vi "Elevator Control PID.vi"(8 "Settings":T4={"min speed"=0.05, "Position Max"=60.0, "gravity"=0.05, "PID Constants"={"P Gain"=0.2, "I Gain"=0.0, "D Gain"=0.2, "F Gain"=0.0, "I Zone"=0.0, "Min Output"=-1.0, "Max Output"=1.0}, "SM Params"={"Max Velocity"=2000.0, "Max Acceleration"=1500.0, "Minimum Velocity Output"=0.0, "Allowed Closed Loop Error"=0.0}} {"gravity" format="%#_13g"; "Position Max" format="%#_13g"; "min speed" format="%#_13g"}, 9 "Manual":bool, 10 "Setpoint":dbl, 11 "Controller In":T6={"Setpoint"=0.0, "Output"=0.0, "DriveMotor1"={"DeviceStatus"={"status"=FALSE, "code"=0, "source"=""}, "Type"=enum."PWM", "PWM"={"PWM Channel"=enum."Invalid", "DeadBand"={"Name"="", "maxPositivePwm"=0, "minPositivePwm"=0, "centerPwm"=0, "maxNegativePwm"=0, "minNegativePwm"=0, "angularRange"=0}}, "CAN"={"Device Number"=0, "SetOutput VI Ref"=variant(enum8{"Percent VBus", "Current", "Speed", "Position", "Voltage"} enum."Percent VBus"), "GetOutput VI Ref"=variant(refnum<k1> refnum), "Enable VI Ref"=variant(dbl 12.0), "Disable VI Ref"=variant(enum8{"Percent VBus", "Speed", "Position", "Slave", "Unchanged / Invalid"} enum."Percent VBus"), "Data"=variant(enum16{"Controller 1"} enum."Controller 1")}, "Invert"=FALSE, "DIO PWM"={"PWM \"Enable\" Channel"=enum."Invalid", "DIOChannel"=enum."Invalid", "PWM Rate"=0.0}}, "Is Done Moving?"=FALSE}) -> (0 "Switches":T3, 1 "Path is Done?":bool, 2 "PID Chart":T2(graph), 3 "Controller out":T6={"Setpoint"=0.0, "Output"=0.0, "DriveMotor1"={"DeviceStatus"={"status"=FALSE, "code"=0, "source"=""}, "Type"=enum."PWM", "PWM"={"PWM Channel"=enum."Invalid", "DeadBand"={"Name"="", "maxPositivePwm"=0, "minPositivePwm"=0, "centerPwm"=0, "maxNegativePwm"=0, "minNegativePwm"=0, "angularRange"=0}}, "CAN"={"Device Number"=0, "SetOutput VI Ref"=variant(enum8{"Percent VBus", "Current", "Speed", "Position", "Voltage"} enum."Percent VBus"), "GetOutput VI Ref"=variant(refnum<k1> refnum), "Enable VI Ref"=variant(dbl 12.0), "Disable VI Ref"=variant(enum8{"Percent VBus", "Speed", "Position", "Slave", "Unchanged / Invalid"} enum."Percent VBus"), "Data"=variant(enum16{"Controller 1"} enum."Controller 1")}, "Invert"=FALSE, "DIO PWM"={"PWM \"Enable\" Channel"=enum."Invalid", "DIOChannel"=enum."Invalid", "PWM Rate"=0.0}}, "Is Done Moving?"=FALSE})   [LabVIEW 2018]
uses:
  Typedef/Controller Data.ctl
  <vilib>/Rock Robotics/WPI/MotorControl/WPI_MotorControlDeviceRef.ctl
  <vilib>/Rock Robotics/WPI/MotorControl/WPI_MotorControlType.ctl
  <vilib>/Rock Robotics/SystemInterfaces/DIO/FPGA_DIOPWMChannel.ctl
  <vilib>/Rock Robotics/WPI/PWM/WPI_PWMDeadband.ctl
  <vilib>/Rock Robotics/SystemInterfaces/DIO/FPGA_DIOChannel.ctl
  Typedef/Elevator Settings.ctl
  <vilib>/Rock Robotics/WPI/ThirdParty/REV Robotics/SPARK MAX/Typedef/Spark MAX Smart Motion Parameters.ctl
  <vilib>/Rock Robotics/WPI/ThirdParty/REV Robotics/SPARK MAX/Typedef/Spark MAX Control Type.ctl
panel:
  out "Waveform Chart":T1(graph)
  # "s"
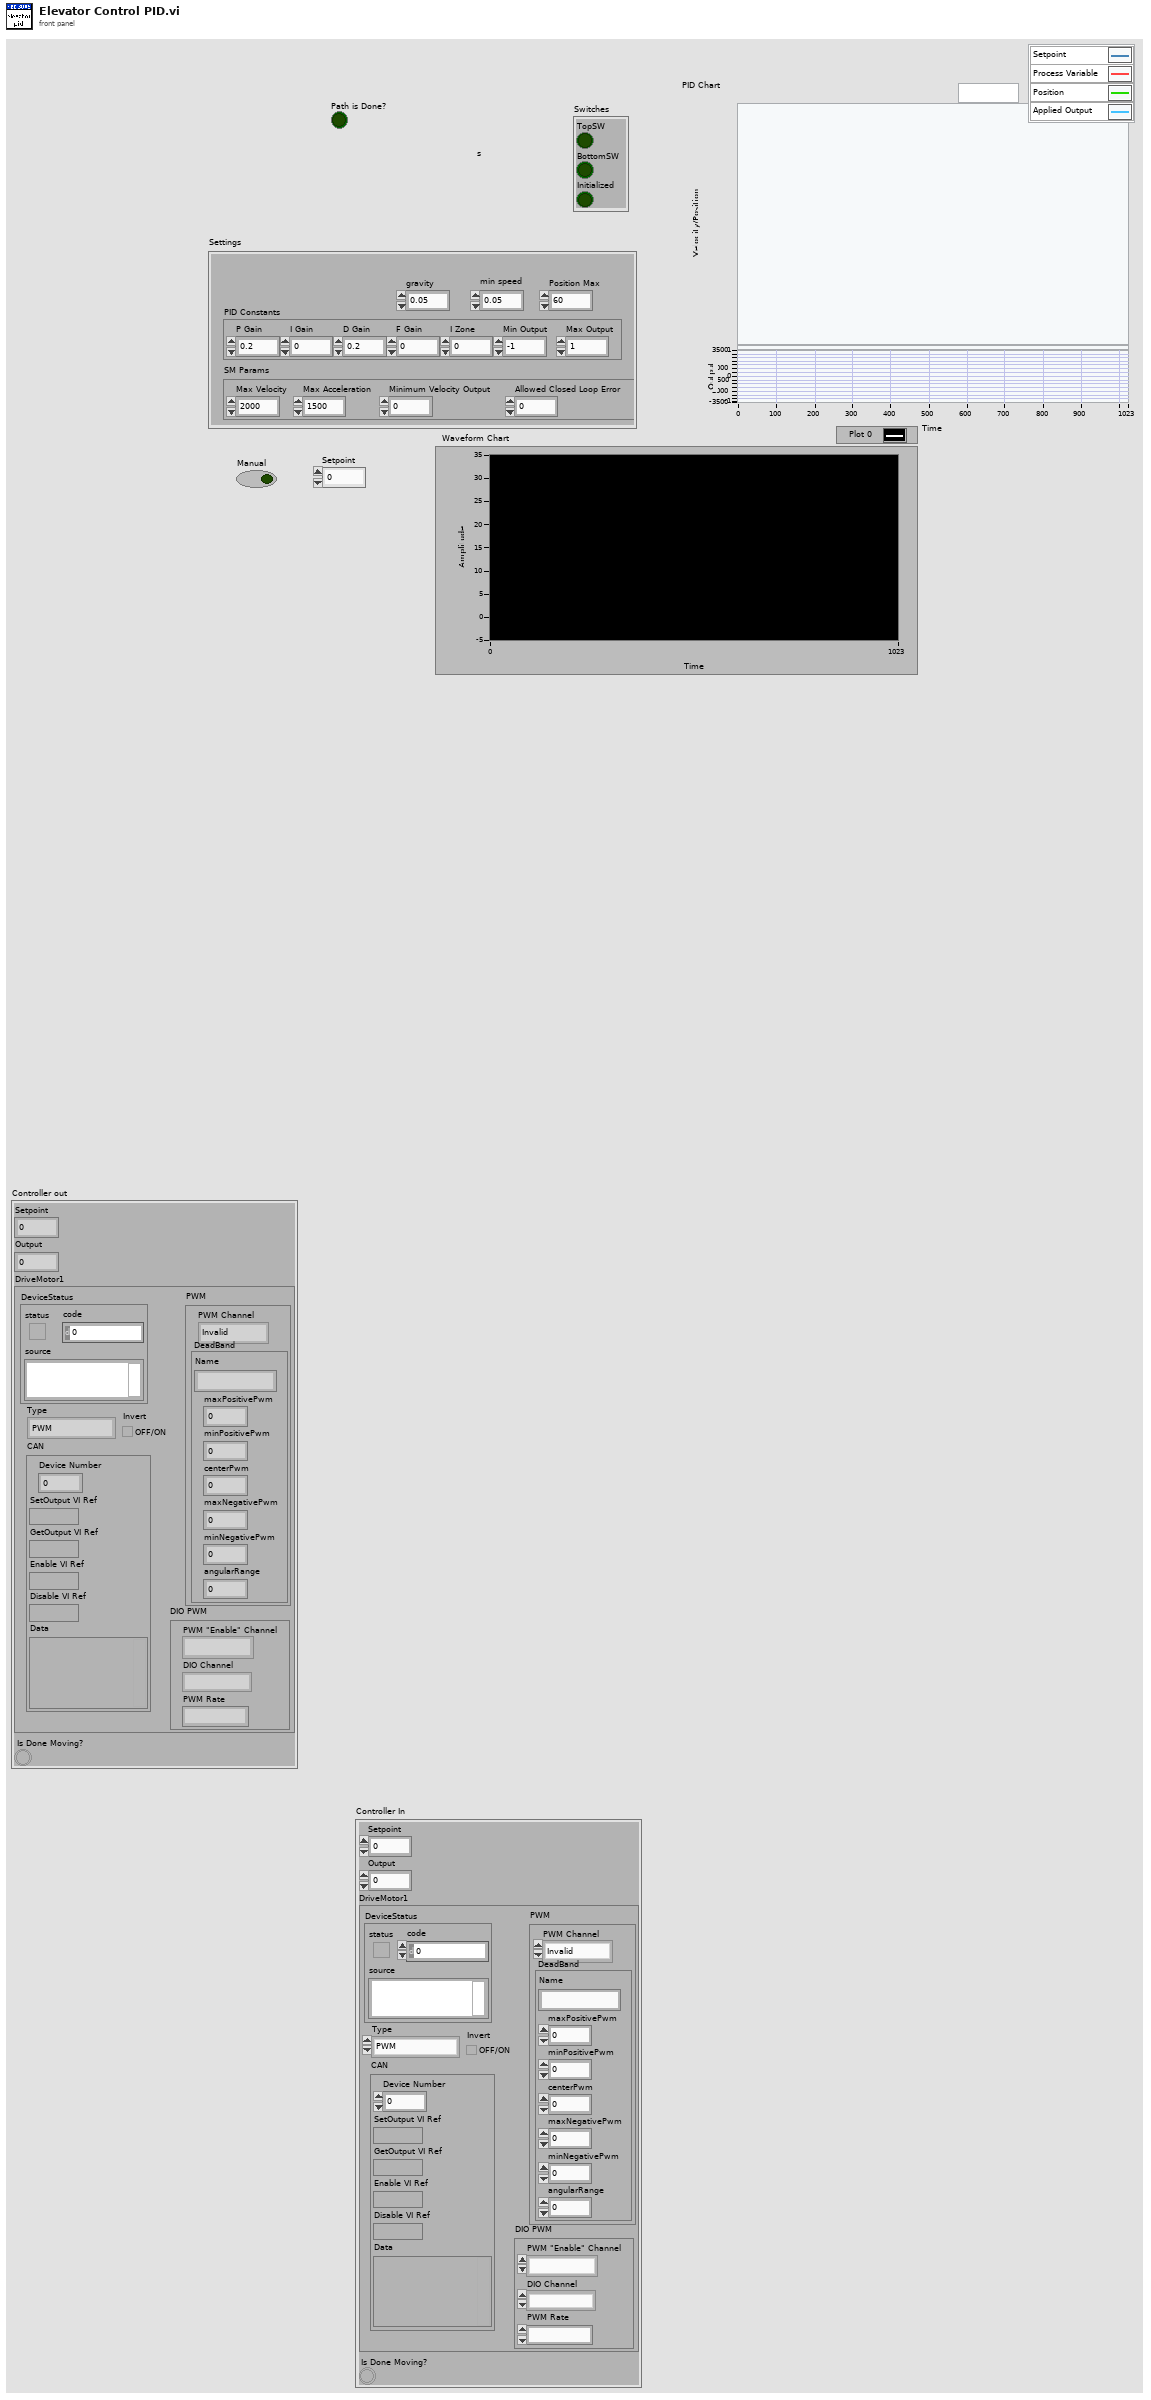
[diagram p1: front panel]
types:
  T1 = cluster{"Sensor Position":dbl, "Sensor Position":dbl}
  T2 = cluster{"Sensor Velocity":dbl, "Setpoint":dbl, "Sensor Position":dbl, "Applied Output":dbl}
  T3 = cluster{"TopSW":bool, "BottomSW":bool, "Initialized":bool}
  T4 = typedef "Elevator Settings.ctl" = cluster{"min speed":dbl, "Position Max":dbl, "gravity":dbl, "PID Constants":cluster{"P Gain":dbl, "I Gain":dbl, "D Gain":dbl, "F Gain":dbl, "I Zone":dbl, "Min Output":dbl, "Max Output":dbl}, "SM Params":T5}
  T5 = typedef "Spark MAX Smart Motion Parameters.ctl" = cluster{"Max Velocity":dbl, "Max Acceleration":dbl, "Minimum Velocity Output":dbl, "Allowed Closed Loop Error":dbl}
  T6 = typedef "Controller Data.ctl" = cluster{"Setpoint":dbl, "Output":dbl, "DriveMotor1":T7, "Is Done Moving?":bool}
  T7 = typedef "WPI_MotorControlDeviceRef.ctl" = cluster{"DeviceStatus":errorcluster, "Type":T8, "PWM":cluster{"PWM Channel":T9, "DeadBand":T10}, "CAN":cluster{"Device Number":u8, "SetOutput VI Ref":variant, "GetOutput VI Ref":variant, "Enable VI Ref":variant, "Disable VI Ref":variant, "Data":variant}, "Invert":bool, "DIO PWM":cluster{"PWM \"Enable\" Channel":T9, "DIOChannel":T11, "PWM Rate":dbl}}
  T8 = typedef "WPI_MotorControlType.ctl" = enum16{"PWM", "CAN", "DIO PWM"}
  T9 = typedef "FPGA_DIOPWMChannel.ctl" = enum8{"PWM 0", "PWM 1", "PWM 2", "PWM 3", "PWM 4", "PWM 5", "PWM 6", "PWM 7", "PWM 8", "PWM 9", "PWM MXP 0", "PWM MXP 1", "PWM MXP 2", "PWM MXP 3", "PWM MXP 4", "PWM MXP 5", "PWM MXP 6", "PWM MXP 7", "PWM MXP 8", "PWM MXP 9", "Invalid"}
  T10 = typedef "WPI_PWMDeadband.ctl" = cluster{"Name":string, "maxPositivePwm":i32, "minPositivePwm":i32, "centerPwm":i32, "maxNegativePwm":i32, "minNegativePwm":i32, "angularRange":u16}
  T11 = typedef "FPGA_DIOChannel.ctl" = enum8{"DIO 0", "DIO 1", "DIO 2", "DIO 3", "DIO 4", "DIO 5", "DIO 6", "DIO 7", "DIO 8", "DIO 9", "DIO MXP 0", "DIO MXP 1", "DIO MXP 2", "DIO MXP 3", "DIO MXP 4", "DIO MXP 5", "DIO MXP 6", "DIO MXP 7", "DIO MXP 8", "DIO MXP 9", "DIO MXP 10", "DIO MXP 11", "DIO MXP 12", "DIO MXP 13", "DIO MXP 14", "DIO MXP 15", "SPI Port CS1", "SPI Port CS2", "SPI Port CS3", "SPI Port MISO", "SPI Port MOSI", "Invalid"}
  T12 = typedef "Spark MAX Control Type.ctl" = enum16{"Percent VBus", "Voltage", "Velocity", "Position", "Smart Motion", "Current", "Smart Velocity"}
  T13 = cluster{"P Gain":dbl, "I Gain":dbl, "D Gain":dbl, "F Gain":dbl, "I Zone":dbl, "Min Output":dbl, "Max Output":dbl}
  T14 = cluster{"P Gain":bool, "I Gain":bool, "D Gain":bool, "F Gain":bool, "I Zone":bool, "Min Output":bool, "Max Output":bool}
  T15 = cluster{"Max Velocity":bool, "Max Acceleration":bool, "Minimum Velocity Output":bool, "Allowed Closed Loop Error":bool}
  T16 = cluster{"Sensor Velocity":dbl, "Position Max":dbl, "Sensor Position":dbl, "Applied Output":dbl}
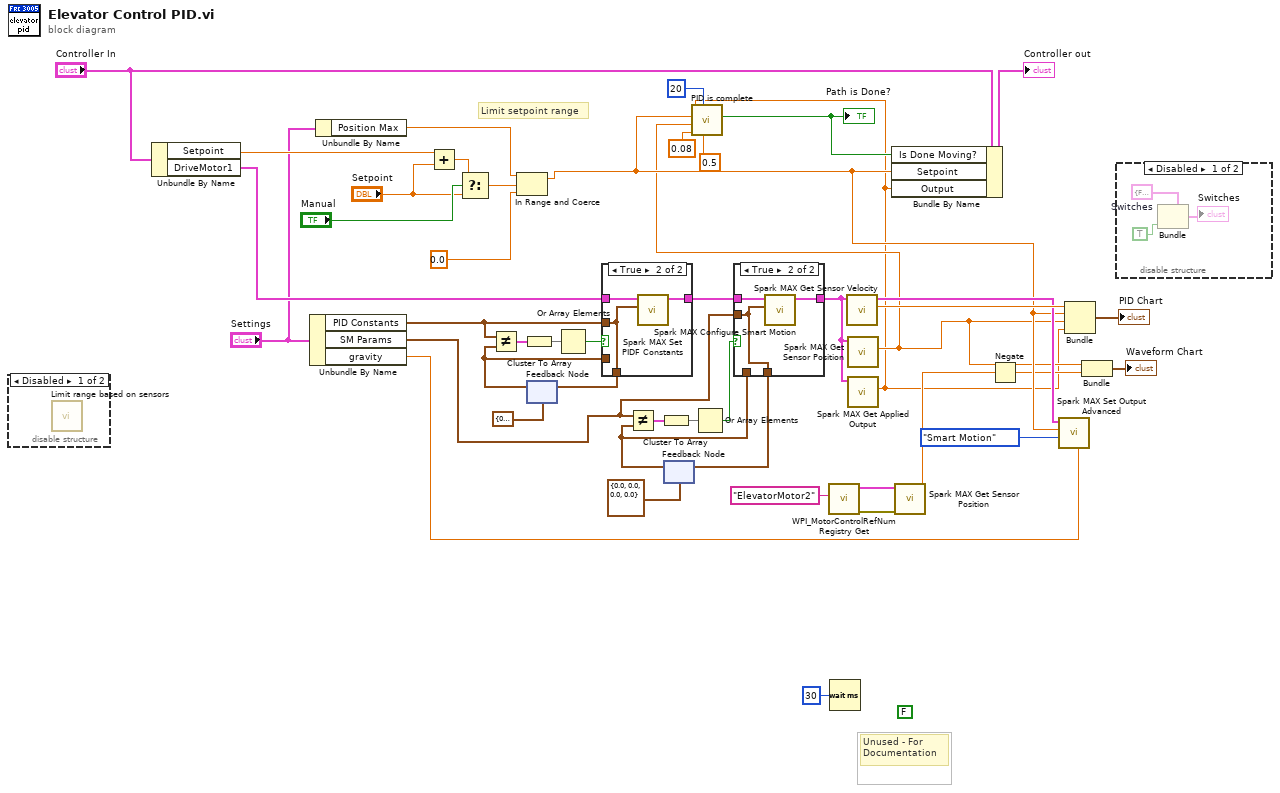
[diagram p0: block diagram]
diagram:
  (unwired) FALSE
  # "Unused - For Documentation"
  # "Limit setpoint range"
  n1 = disable-structure shown="Disabled" {
    frame Disabled {
      n2 = call "Limit range based on sensors.vi"() -> ()  [unwired: 10 in, 2 out]
    }
    frame Enabled {
    }
  }
  n3 = Unbundle By Name("Controller In") -> ("Setpoint"=w46:dbl, "DriveMotor1"=w17:T7)
  n4 = Unbundle By Name("Settings") -> ("PID Constants"=w18:T13, "SM Params"=w16:T5, "gravity"=w13:dbl)
  n5 = Unbundle By Name("Settings") -> ("Position Max"=w11:dbl)
  n6 = Add(x=w46, y="Setpoint") -> (x+y=w41:dbl)
  n7 = Select(t=w41, s="Manual", f="Setpoint") -> (s? t:f=w39:dbl)
  n8 = In Range and Coerce(upper limit=w11, x=w39, lower limit=0.0) -> (coerced(x)=w14:dbl)  [unwired: 1 out]
  n9 = feedback #1(T13 {"P Gain"=0.0, "I Gain"=0.0, "D Gain"=0.0, "F Gain"=0.0, "I Zone"=0.0, "Min Output"=0.0, "Max Output"=0.0} ("PID Constants")) -> (w37:T13)
  n10 = Not Equal?(x=w18, y=w37) -> (x != y?=w32:T14)
  n11 = Cluster To Array(cluster=w32) -> (array=w33:bool[])
  n12 = Or Array Elements(Boolean array=w33) -> (logical OR=w35:bool)
  n13 = case shown="True" w35 {
    tunnel: w17 -> [w47 w51]
    tunnel: w18 -> [_ w49]
    tunnel: [w48 w49] -> w36
    tunnel: w37 -> [w48 _]
    tunnel: [w47 w50] -> w29
    frame False {
    }
    frame True {
      n14 = call <vilib>:"Spark MAX Set PIDF Constants.vi"("PID Constants"=w49, "MotorControlDeviceRef"=w51) -> ("MotorControlDeviceRef"=w50:T7)  [unwired: 8 in, 1 out]
    }
  }
  n15 = feedback-in #1(w36) -> ()
  n16 = feedback #2(T5 {"Max Velocity"=0.0, "Max Acceleration"=0.0, "Minimum Velocity Output"=0.0, "Allowed Closed Loop Error"=0.0} ("Smart Motion Parameters")) -> (w23:T5)
  n17 = Not Equal?(x=w16, y=w23) -> (x != y?=w27:T15)
  n18 = Cluster To Array(cluster=w27) -> (array=w28:bool[])
  n19 = Or Array Elements(Boolean array=w28) -> (logical OR=w26:bool)
  n20 = case shown="True" w26 {
    tunnel: w29 -> [w53 w56]
    tunnel: w16 -> [_ w54]
    tunnel: [w53 w55] -> w20
    tunnel: [w52 w54] -> w24
    tunnel: w23 -> [w52 _]
    frame False {
    }
    frame True {
      n21 = call <vilib>:"Spark MAX Configure Smart Motion.vi"("Smart Motion Parameters"=w54, "MotorControlDeviceRef"=w56) -> ("MotorControlDeviceRef"=w55:T7)  [unwired: 8 in, 1 out]
    }
  }
  n22 = feedback-in #2(w24) -> ()
  n23 = call <vilib>:"WPI_MotorControlRefNum Registry Get.vi"("refnum name"="ElevatorMotor2") -> ("error out"=w6:errorcluster, "MotorControlDevRef"=w5:T7)  [unwired: 9 in]
  n24 = Wait (ms)(milliseconds to wait=u32 30) -> ()  [unwired: 1 out]
  n25 = call <vilib>:"Spark MAX Get Sensor Velocity.vi"("MotorControlDevRef in"=w20) -> ("Sensor Velocity"=w30:dbl, "MotorControlDevRef out"=w21:T7)  [unwired: 7 in, 2 out]
  n26 = call <vilib>:"Spark MAX Get Sensor Position.vi"("MotorControlDevRef in"=w20) -> ("Sensor Position"=w9:dbl)  [unwired: 7 in, 3 out]
  n27 = call <vilib>:"Spark MAX Get Applied Output.vi"("MotorControlDevRef in"=w20) -> ("Applied Output"=w2:dbl)  [unwired: 7 in, 3 out]
  n28 = call "PID is complete.vi"("Error Threshold"=0.5, "sample length"=20, "threshold"=0.08, "process variable"=w9, "setpoint"=w14, "PID Output"=w2) -> ("PID is Done?"=w43:bool)  [unwired: 4 in, 1 out]
  "Path is Done?" <- w43
  n29 = Bundle By Name(cluster="Controller In", "Is Done Moving?"=w43, "Setpoint"=w14, "Output"=w2) -> (→"Controller out":T6)
  n30 = call <vilib>:"Spark MAX Get Sensor Position.vi"("error in (no error)"=w6, "MotorControlDevRef in"=w5) -> ("Sensor Position"=w7:dbl)  [unwired: 6 in, 3 out]
  n31 = Negate(x=w7) -> (-x=w3:dbl)
  n32 = call <vilib>:"Spark MAX Set Output Advanced.vi"("Arbitrary Feed Forward (0)"=w13, "Control Mode"=Spark_MAX_Control_Type."Smart Motion", "Setpoint"=w14, "MotorControlDevRef"=w21) -> ()  [unwired: 6 in, 2 out]
  n33 = Bundle("Sensor Velocity"=w30, "Position Max"=w14, "Sensor Position"=w9, "Applied Output"=w2) -> (→"PID Chart":T16)  [unwired: 1 in]
  n34 = Bundle("Sensor Position"=w9, w3) -> (→"Waveform Chart":cluster{"Sensor Position":dbl, dbl})  [unwired: 1 in]
  n35 = disable-structure shown="Disabled" {
    frame Disabled {
      w59 = T3 {"TopSW"=FALSE, "BottomSW"=FALSE, "Initialized"=FALSE}  # Switches
      n36 = Bundle(cluster=w59, "Initialized"=TRUE) -> (→"Switches":T3)  [unwired: 2 in]
    }
    frame Enabled {
    }
  }
